vi "set_up_graph_hardware_window_properties.vi"(9 "Graph Properties":T1, 11 "Hardware Window Refnum":refnum<vi>) -> ()   [LabVIEW 2017, in "3DPC_SurfacePlot.xctl"]
uses:
  <vilib>/Native 3D Graph/xcontrol/3DPC_SurfacePlot.xctl
  <vilib>/Native 3D Graph/typedefs/prop_graph.ctl
  <vilib>/picture/3D Picture Control/NI_3D Picture Control.lvlib
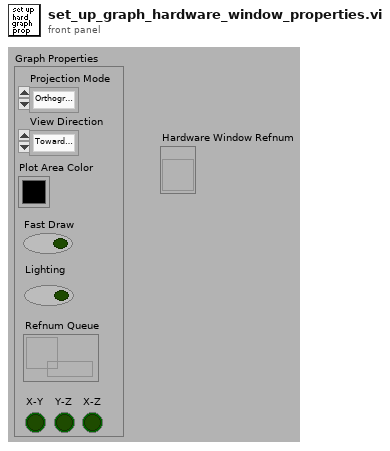
[diagram p1: front panel]
types:
  T1 = typedef "3DPC_SurfacePlot.xctl/prop_graph.ctl" = cluster{"Projection Mode":enum16{"Orthographic", "Perspective"}, "View Direction":enum32{"Towards X-Y Plane", "Towards Y-Z Plane", "Towards X-Z Plane", "User Define"}, "Plot Area Color":u32, "Fast Draw":bool, "X-Y":bool, "Y-Z":bool, "X-Z":bool, "Lighting":bool, "Refnum Queue":refnum<queue>}
  T2 = enum32{"Towards X-Y Plane", "Towards Y-Z Plane", "Towards X-Z Plane", "User Define"}
  T3 = enum16{"None", "Spherical", "Flying", "Oriented"}
  T4 = cluster{"Left":sgl, "Left":sgl, "Left":sgl, "Left":sgl, "Left":sgl, "Left":sgl}
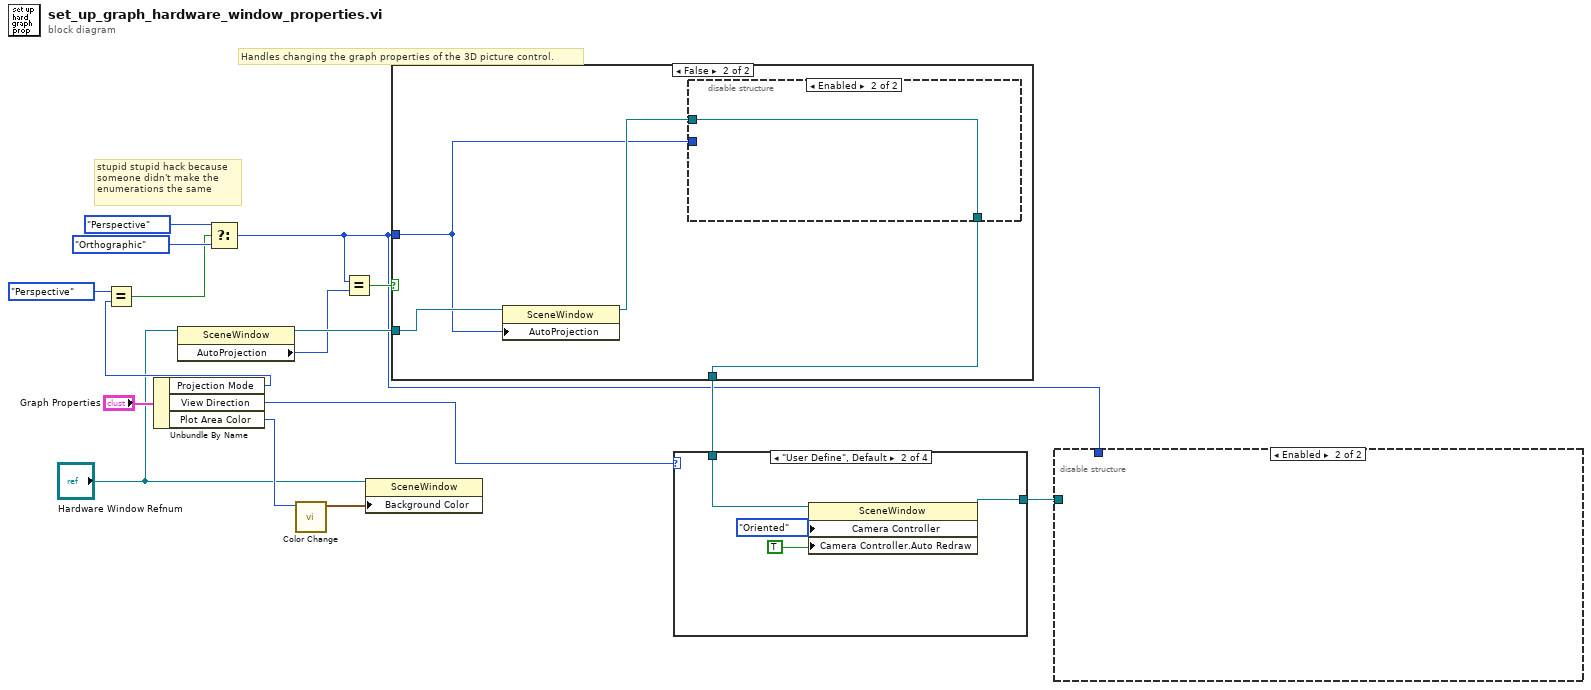
[diagram p0: block diagram]
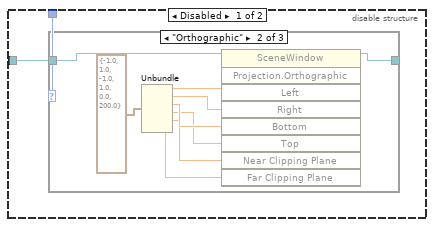
[diagram p2: hidden frame]
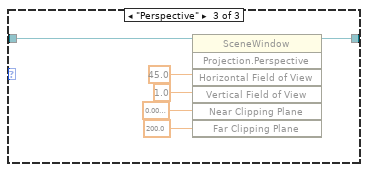
[diagram p4: hidden frame]
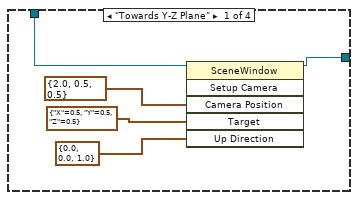
[diagram p5: hidden frame]
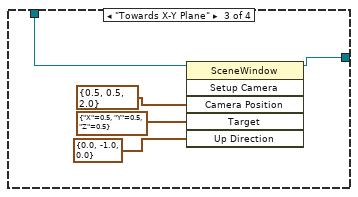
[diagram p6: hidden frame]
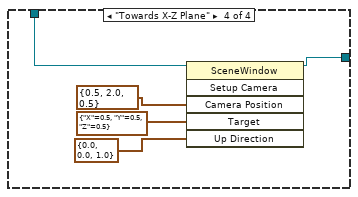
[diagram p7: hidden frame]
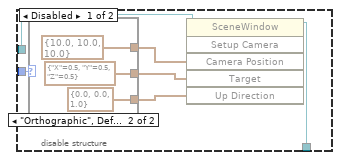
[diagram p9: hidden frame]
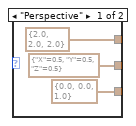
[diagram p10: hidden frame]
diagram:
  # "stupid stupid hack because\nsomeone didn't make the \nenumerations the same"
  # "Handles changing the graph properties of the 3D picture control."
  n1 = Unbundle By Name("Graph Properties") -> ("Projection Mode"=w7:enum16{"Orthographic", "Perspective"}, "View Direction"=w15:T2, "Plot Area Color"=w14:u32)
  n2 = Equal?(x=enum16{"Orthographic", "Perspective"}."Perspective", y=w7) -> (x = y?=w5:bool)
  n3 = property class="SceneWindow"(reference="Hardware Window Refnum") -> (reference out=w11:refnum<vi>, "AutoProjection"=w2:enum16{"None", "Perspective", "Orthographic"})  [unwired: 1 in, 1 out]
  n4 = Select(t=enum16{"None", "Perspective", "Orthographic"}."Perspective" ("Automatic Projection Mode"), s=w5, f=enum16{"None", "Perspective", "Orthographic"}."Orthographic" ("Automatic Projection Mode")) -> (s? t:f=w1:enum16{"None", "Perspective", "Orthographic"})
  n5 = call <vilib>:"Color Change.vi"("Color"=w14) -> ("RGBA"=w13:cluster{"R":sgl, "G":sgl, "B":sgl, "A":sgl})  [unwired: 1 in, 9 out]
  n6 = Equal?(x=w1, y=w2) -> (x = y?=w12:bool)
  n7 = property on="Property Node" class="SceneWindow"(reference="Hardware Window Refnum", "Background Color"=w13) -> ()  [unwired: 1 in, 2 out]
  n8 = case shown="False" w12 {
    tunnel: [w17 w18] -> w10
    tunnel: w11 -> [w17 w21]
    tunnel: w1 -> [_ w19]
    frame True {
    }
    frame False {
      n9 = property class="SceneWindow"(reference=w21, "AutoProjection"=w19) -> (reference out=w20:refnum<vi>)  [unwired: 1 in, 1 out]
      n10 = disable-structure shown="Enabled" {
        disable-tunnel: w20 -> [w24 w34]
        disable-tunnel: w19 -> [w23 _]
        disable-tunnel: [w22 w34] -> w18
        frame Disabled {
          n11 = case shown="\"Orthographic\", Default" w23 {
            tunnel: [cluster{"Z":sgl, "Y":sgl, "X":sgl} {"Z"=0.0, "Y"=0.0, "X"=1.0} cluster{"Z":sgl, "Y":sgl, "X":sgl} {"Z"=0.0, "Y"=0.0, "X"=1.0}] -> w27
            tunnel: [cluster{"X":sgl, "Y":sgl, "Z":sgl} {"X"=0.5, "Y"=0.5, "Z"=0.5} ("Target") cluster{"X":sgl, "Y":sgl, "Z":sgl} {"X"=0.5, "Y"=0.5, "Z"=0.5} ("Target")] -> w26
            tunnel: [cluster{"X":sgl, "Y":sgl, "Z":sgl} {"X"=2.0, "Y"=2.0, "Z"=2.0} ("Up Direction") cluster{"X":sgl, "Y":sgl, "Z":sgl} {"X"=10.0, "Y"=10.0, "Z"=10.0} ("Up Direction")] -> w25
            frame "Perspective" {
            }
            frame "Orthographic", Default {
            }
          }
          n12 = invoke on="Invoke Node" class="SceneWindow" method="Setup Camera"(reference=w24, "Camera Position"=w25, "Target"=w26, "Up Direction"=w27) -> (reference out=w22:refnum<vi>)  [unwired: 2 in, 5 out]
        }
        frame Enabled {
        }
      }
    }
  }
  n13 = case shown="\"User Define\", Default" w15 {
    tunnel: w10 -> [w36 w42 w45 w50]
    tunnel: [w35 w40 w44 w49] -> w3
    frame "Towards Y-Z Plane" {
      n14 = invoke class="SceneWindow" method="Setup Camera"(reference=w36, "Camera Position"=cluster{"X":sgl, "Y":sgl, "Z":sgl} {"X"=2.0, "Y"=0.5, "Z"=0.5}, "Target"=cluster{"X":sgl, "Y":sgl, "Z":sgl} {"X"=0.5, "Y"=0.5, "Z"=0.5} ("Camera Position"), "Up Direction"=cluster{"X":sgl, "Y":sgl, "Z":sgl} {"X"=0.0, "Y"=0.0, "Z"=1.0} ("Camera Position")) -> (reference out=w35:refnum<vi>)  [unwired: 2 in, 5 out]
    }
    frame "User Define", Default {
      n15 = property class="SceneWindow"(reference=w42, "Camera Controller"=T3."Oriented" ("Camera Controller:Type"), "Camera Controller.Auto Redraw"=TRUE ("Camera Controller:Auto Redraw")) -> (reference out=w40:refnum<vi>)  [unwired: 1 in, 1 out]
    }
    frame "Towards X-Y Plane" {
      n16 = invoke class="SceneWindow" method="Setup Camera"(reference=w45, "Camera Position"=cluster{"X":sgl, "Y":sgl, "Z":sgl} {"X"=0.5, "Y"=0.5, "Z"=2.0}, "Target"=cluster{"X":sgl, "Y":sgl, "Z":sgl} {"X"=0.5, "Y"=0.5, "Z"=0.5} ("Camera Position"), "Up Direction"=cluster{"X":sgl, "Y":sgl, "Z":sgl} {"X"=0.0, "Y"=-1.0, "Z"=0.0} ("Camera Position")) -> (reference out=w44:refnum<vi>)  [unwired: 2 in, 5 out]
    }
    frame "Towards X-Z Plane" {
      n17 = invoke class="SceneWindow" method="Setup Camera"(reference=w50, "Camera Position"=cluster{"X":sgl, "Y":sgl, "Z":sgl} {"X"=0.5, "Y"=2.0, "Z"=0.5}, "Target"=cluster{"X":sgl, "Y":sgl, "Z":sgl} {"X"=0.5, "Y"=0.5, "Z"=0.5} ("Camera Position"), "Up Direction"=cluster{"X":sgl, "Y":sgl, "Z":sgl} {"X"=0.0, "Y"=0.0, "Z"=1.0} ("Camera Position")) -> (reference out=w49:refnum<vi>)  [unwired: 2 in, 5 out]
    }
  }
  n18 = disable-structure shown="Enabled" {
    disable-tunnel: w3 -> [w55 _]
    disable-tunnel: w1 -> [w54 _]
    frame Disabled {
      n19 = case shown="\"Orthographic\"" w54 {
        tunnel: w55 -> [w56 w58 w67]
        tunnel: [w56 w57 w66] -> _
        frame "None", Default {
        }
        frame "Orthographic" {
          n20 = Unbundle(T4 {"Left"=-1.0, "Left"=1.0, "Left"=-1.0, "Left"=1.0, "Left"=0.0, "Left"=200.0} ("output cluster")) -> ("Left"=w64:sgl, "Left"=w63:sgl, "Left"=w62:sgl, "Left"=w61:sgl, "Left"=w60:sgl, "Left"=w59:sgl)
          n21 = invoke on="Invoke Node" class="SceneWindow" method="Projection.Orthographic"(reference=w58, "Left"=w64, "Right"=w63, "Bottom"=w62, "Top"=w61, "Near Clipping Plane"=w60, "Far Clipping Plane"=w59) -> (reference out=w57:refnum<vi>)  [unwired: 2 in, 8 out]
        }
        frame "Perspective" {
          n22 = invoke on="Invoke Node" class="SceneWindow" method="Projection.Perspective"(reference=w67, "Horizontal Field of View"=sgl 45.0 ("Field of View"), "Vertical Field of View"=sgl 1.0 ("Aspect Ratio"), "Near Clipping Plane"=sgl 0.01, "Far Clipping Plane"=sgl 200.0) -> (reference out=w66:refnum<vi>)  [unwired: 2 in, 6 out]
        }
      }
    }
    frame Enabled {
    }
  }
